vi "Qnet_Globals.vi"() -> ()   [LabVIEW 2010]
uses:
  Controls/HTML_Section_Cluster.ctl
panel:
  in  "Section Clusters":T1[](array[typedef])
  in  "border-right":string="border-right:1.5pt solid black;"
  in  "border-left":string="border-left:1.5pt solid black;"
  in  "border-bottom":string="border-bottom:1.5pt solid black;"
  in  "border-top":string="border-top:1.5pt solid black;"
  in  "Index Sheet End 2":string="</table>\n</td>\n</tr>\n</div>\n</table>\n</body>\n\n</html>\n\n"
  in  "Local Site Root":path=path "Please Run EnFlo Hub.vi"
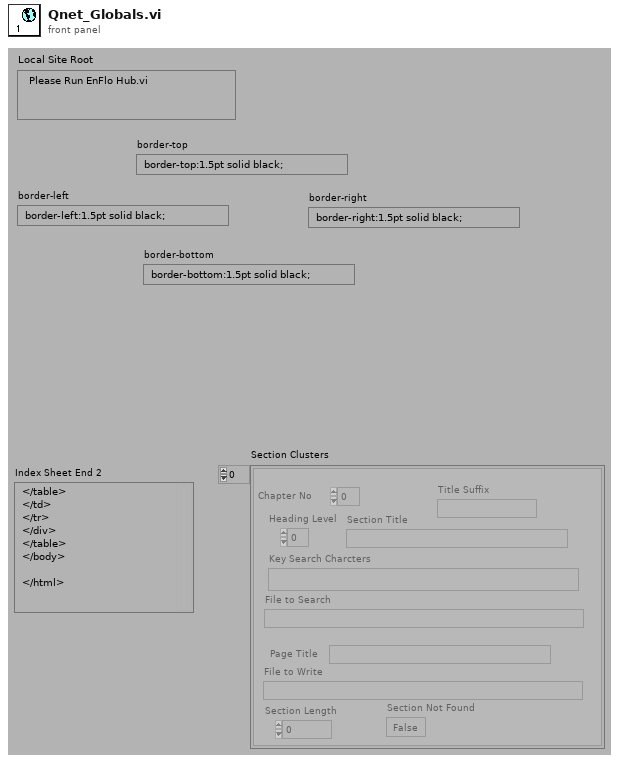
[diagram p1: front panel]
types:
  T1 = typedef "HTML_Section_Cluster.ctl" = cluster{"Chapter No":i32, "Heading Level":i32, "Section Title":string, "Key Search Charcters":string, "File to Search":path, "File to Write":path, "Page Title":string, "Section Length":i32, "Section Not Found":bool, "Title Suffix":string}
diagram:
